vi "Rinocloud_explorer_v0.2.vi"() -> ()   [LabVIEW 2013]
uses:
  Rinocloud_global_variable.vi
panel:
  in  "Extra metadata array":T1(array[cluster])=[{"Attribute"="", "Value"="", "Data type"=enum."<null>"}]
  in  "source ID":string
  in  "destination ID":string
  out "error out":errorcluster
  in  "Active item:":string
  out "RId:":string
  out "OId:":string
  out "FId:":string
  out "DId:":string
  in  "delete":bool
  in  "refresh list":bool
  in  "Tab Control":T2(tab)
  in  "Cluster 2":T3={"Attribute"="Amplitude", "Value"="10", "Data type"=5} {"Data type" items=["Numeric", "String", "1D array of strings", "1D array of doubles", "Data JSON string", "<null>"]}
  in  "Cluster 1":T3={"Attribute"="Amplitude", "Value"="10", "Data type"=5} {"Data type" items=["Numeric", "String", "1D array of strings", "1D array of doubles", "Data JSON string", "<null>"]}
  in  "name":string
  in  "tags":string
  in  "notes":string
  in  "new folder":bool
  in  "upload file":bool
  in  "Name:":string
  in  "Tags:":string
  in  "Notes:":string
  in  "get metadata":bool
  in  "metadata tree":string(tree) caption="Metadata"
  in  "update metadata":bool
  in  "Move":bool
  in  "Destination:":string
  in  "Source:":string
  in  "set source":bool
  in  "set destination":bool
  out "body":string
  out "headers":string
  in  "Active object ID":string
  in  "Active file ID":string
  in  "Active dir ID":string
  in  "Recent ID":string
  in  "menu tree":string(tree) caption="Active path"
  in  "stop":bool
  in  "active child tree":string(tree) caption="File & folder list of the active folder"
  # "Double-click an item to activate"
  # "Custom metadata:"
  # "(tag1,tag2,tag3,...)"
  # "Click the fields to edit"
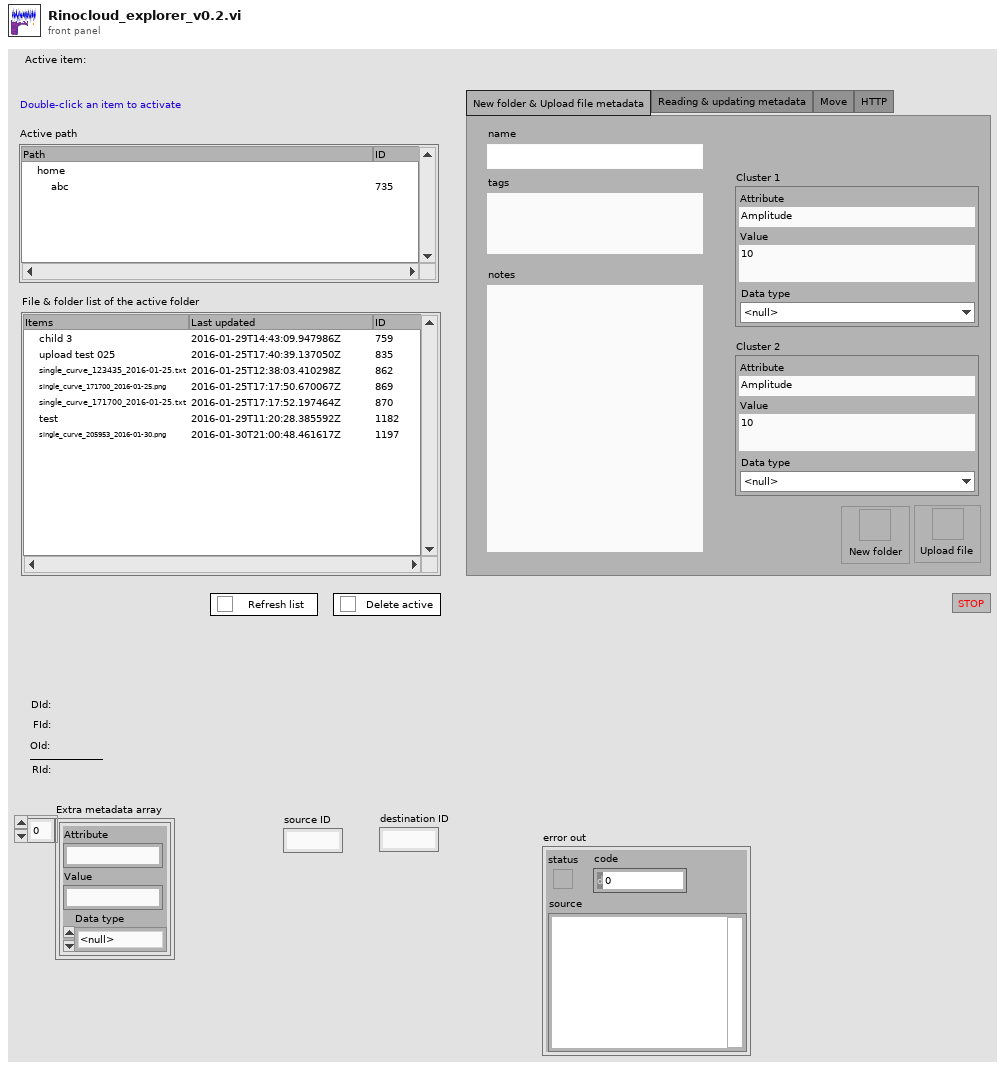
[diagram p1: front panel]
types:
  T1 = cluster{"Attribute":string, "Value":string, "Data type":enum16{"Numeric", "String", "1D array of strings", "1D array of doubles", "Data JSON string", "<null>"}}[]
  T2 = enum32{"New folder & Upload file metadata", "Reading & updating metadata", "Move", "HTTP"}
  T3 = cluster{"Attribute":string, "Value":string, "Data type":u16}
  T4 = cluster{"headers":string, "body":string, "ID":string, "Saved":bool}
  T5 = cluster{"Attribute":string, "Value":string, "Data type":u16}[]
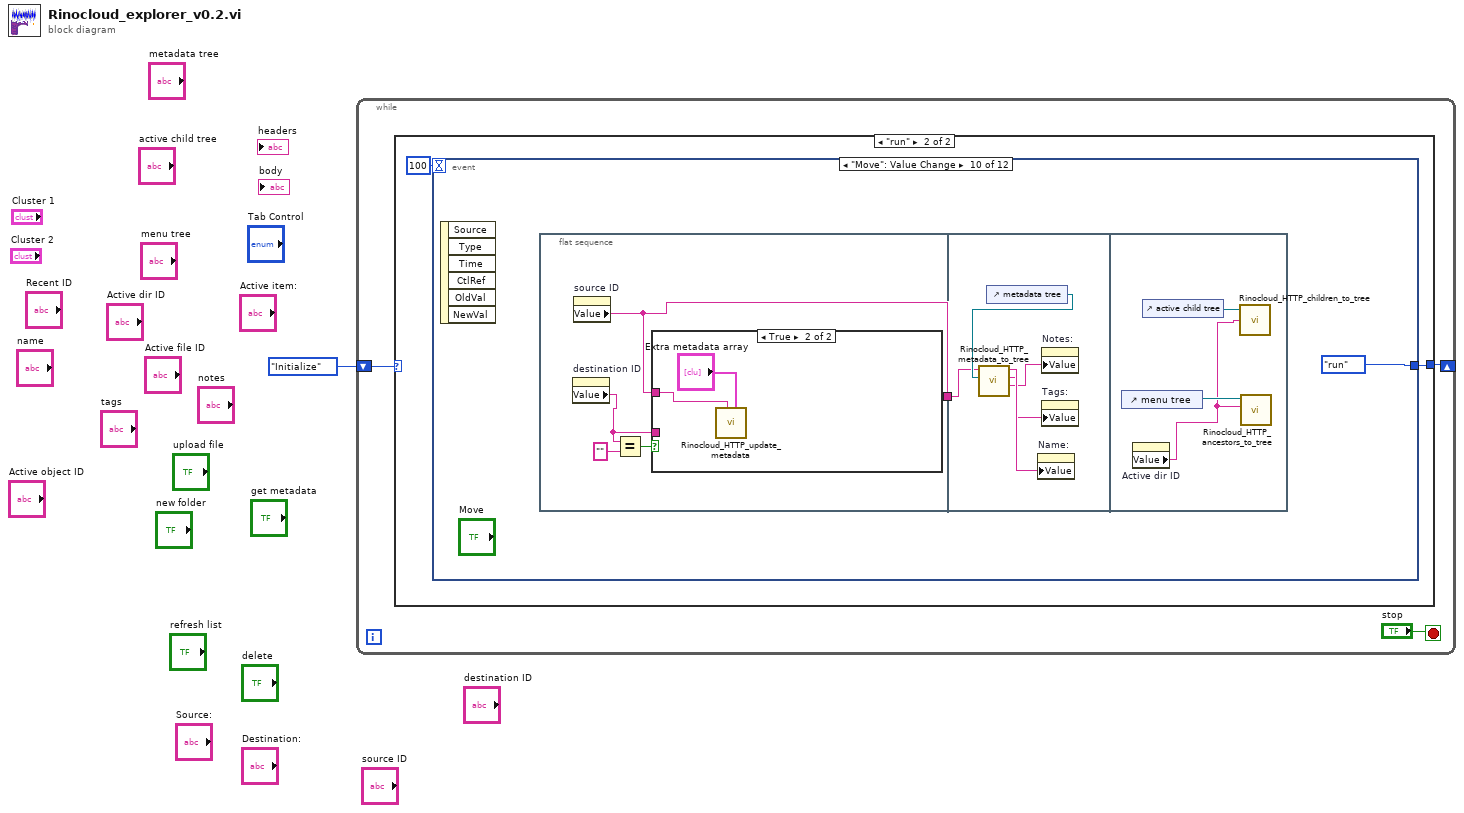
[diagram p0: block diagram]
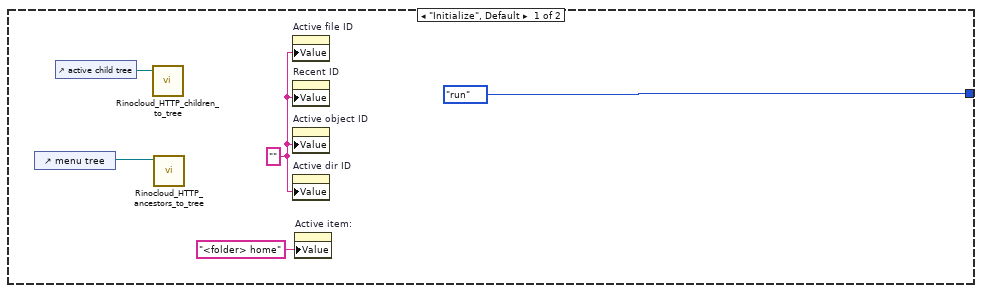
[diagram p2: hidden frame]
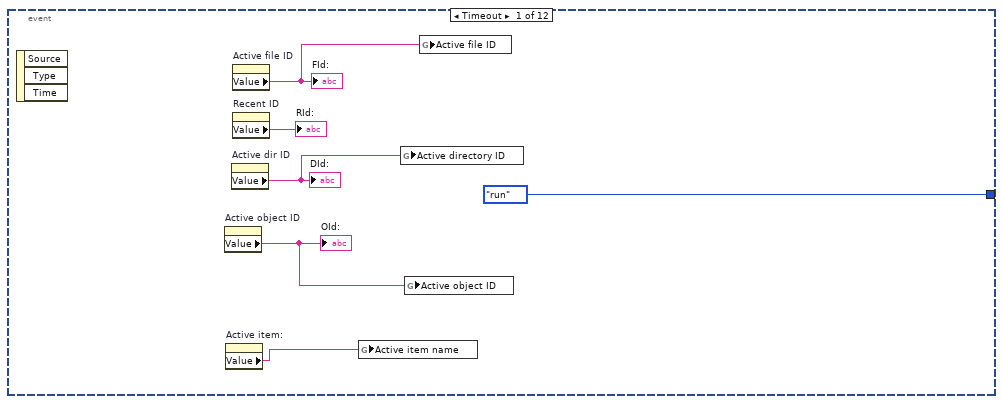
[diagram p3: hidden frame]
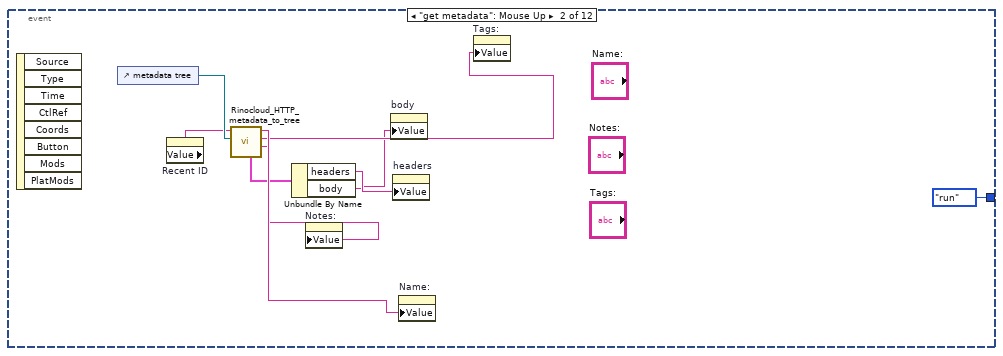
[diagram p4: hidden frame]
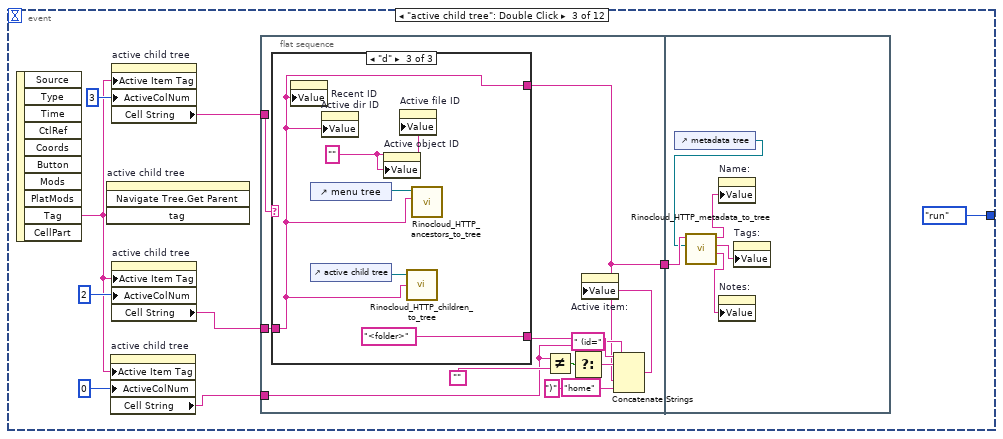
[diagram p5: hidden frame]
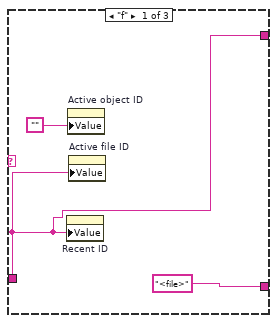
[diagram p6: hidden frame]
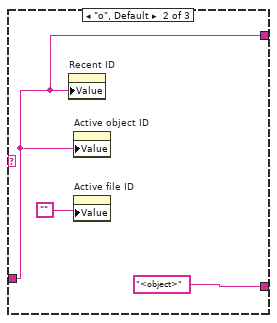
[diagram p7: hidden frame]
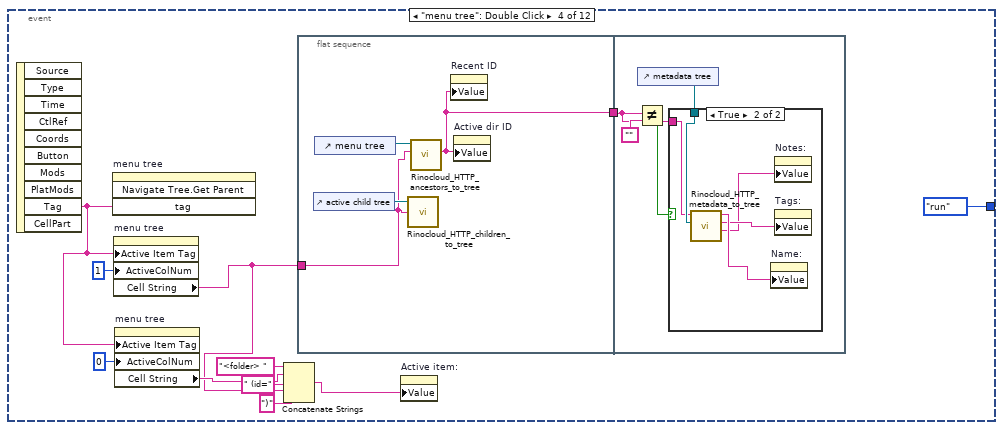
[diagram p8: hidden frame]
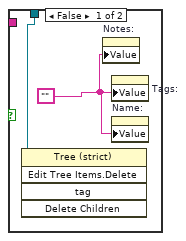
[diagram p9: hidden frame]
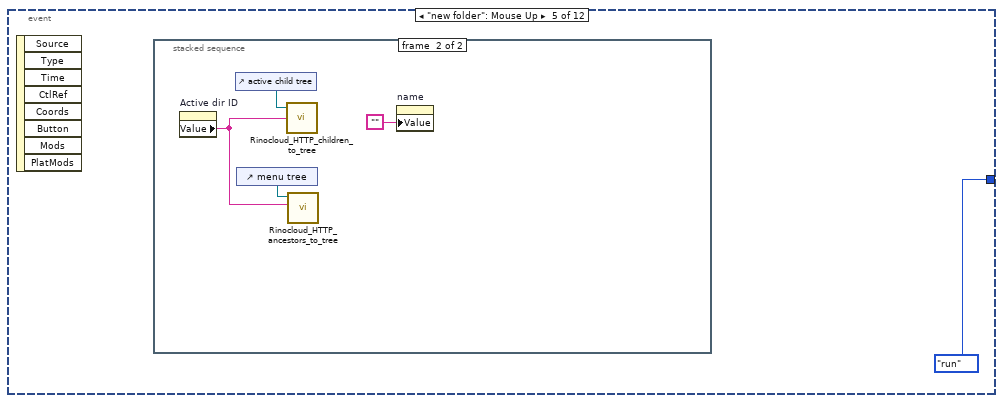
[diagram p10: hidden frame]
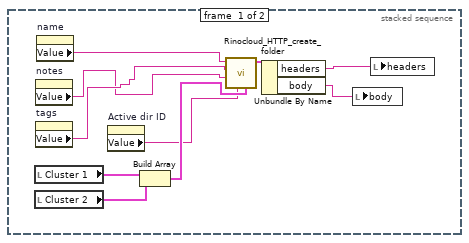
[diagram p11: hidden frame]
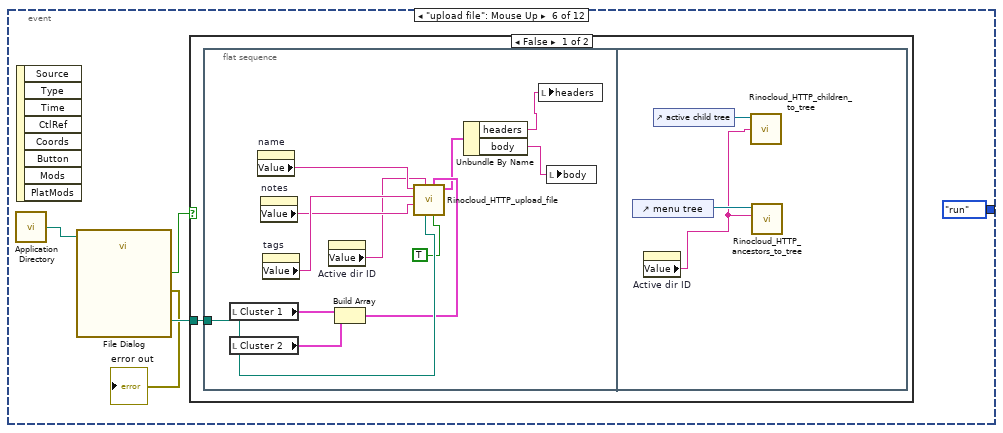
[diagram p12: hidden frame]
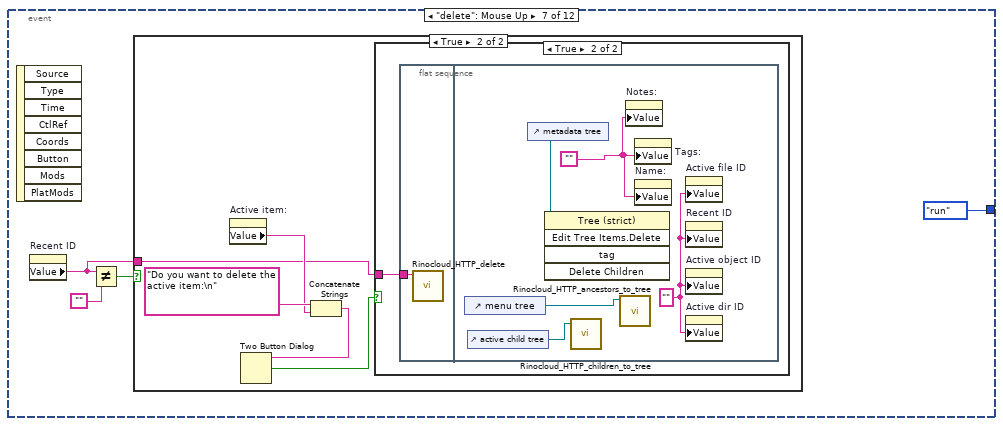
[diagram p14: hidden frame]
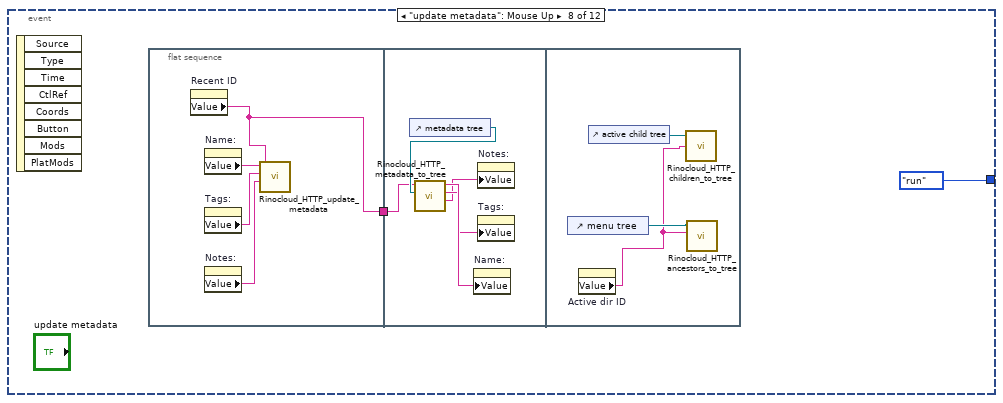
[diagram p17: hidden frame]
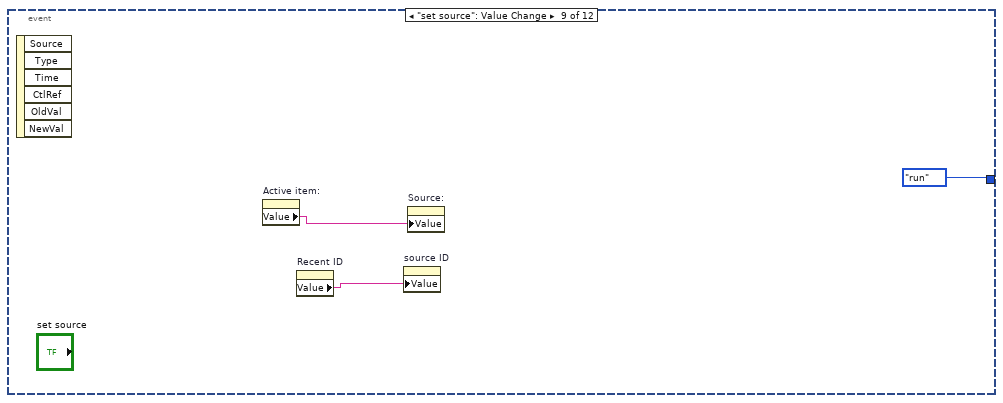
[diagram p18: hidden frame]
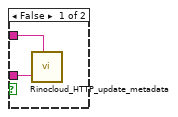
[diagram p19: hidden frame]
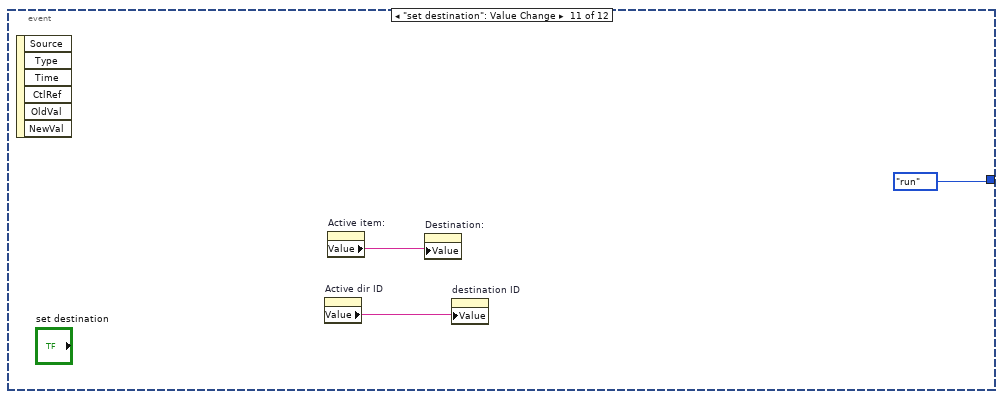
[diagram p20: hidden frame]
diagram:
  n1 = while {
    shift-right: [w3] -> _
    shift-left: enum16{"Initialize"}."Initialize" -> [w4]
    stop <- "stop" stop-if-true
    n2 = case shown="\"run\"" w4 {
      tunnel: [enum16{"Initialize", "run"}."run" w11] -> w3
      frame "Initialize", Default {
        w8 = "" ("Active file ID")
        n3 = control-ref of="menu tree"() -> (w5:refnum<vi>)
        n4 = control-ref of="active child tree"() -> (w6:refnum<vi>)
        n5 = call "Rinocloud_HTTP_children_to_tree.vi"("Tree Ref in"=w6) -> ()  [unwired: 3 in, 2 out]
        n6 = call "Rinocloud_HTTP_ancestors_to_tree.vi"("Tree Ref in"=w5) -> ()  [unwired: 3 in, 4 out]
        n7 = property on="Active file ID" class="Str"("Value"=w8) -> ()  [unwired: 2 in, 2 out]
        n8 = property on="Recent ID" class="Str"("Value"=w8) -> ()  [unwired: 2 in, 2 out]
        n9 = property on="Active object ID" class="Str"("Value"=w8) -> ()  [unwired: 2 in, 2 out]
        n10 = property on="Active dir ID" class="Str"("Value"=w8) -> ()  [unwired: 2 in, 2 out]
        n11 = property on="Active item:" class="Str"("Value"="<folder> home" ("An active item:")) -> ()  [unwired: 2 in, 2 out]
      }
      frame "run" {
        n12 = event shown="[9] \"Move\": Value Change" {
          selector: _ -> [_ _ _ _ _ _ _ _ _ _ _ _]
          dyn-events: _ -> [_ _ _ _ _ _ _ _ _ _ _ _]
          timeout: 100 -> [_ _ _ _ _ _ _ _ _ _ _ _]
          tunnel: [enum16{"Initialize", "run"}."run" enum16{"Initialize", "run"}."run" enum16{"Initialize", "run"}."run" enum16{"Initialize", "run"}."run" enum16{"Initialize", "run"}."run" enum16{"Initialize", "run"}."run" enum16{"Initialize", "run"}."run" enum16{"Initialize", "run"}."run" enum16{"Initialize", "run"}."run" enum16{"Initialize", "run"}."run" enum16{"Initialize", "run"}."run" enum16{"Initialize", "run"}."Initialize"] -> w11
          event Timeout {
            n13 = event-data() -> ()  [unwired: 1 in, 3 out]
            n14 = property on="Active object ID" class="Str"() -> ("Value"=w13:string)  [unwired: 2 in, 2 out]
            "OId:" <- w13
            n15 = property on="Active item:" class="Str"() -> ("Value"=w12:string)  [unwired: 2 in, 2 out]
            n16 = property on="Active dir ID" class="Str"() -> ("Value"=w14:string)  [unwired: 2 in, 2 out]
            "DId:" <- w14
            n17 = property on="Active file ID" class="Str"() -> ("Value"=w15:string)  [unwired: 2 in, 2 out]
            "FId:" <- w15
            n18 = property on="Recent ID" class="Str"() -> ("Value"=→"RId:":string)  [unwired: 2 in, 2 out]
            n19 = global write "Rinocloud_global_variable.vi" "Active item name"(w12) -> ()
            n20 = global write "Rinocloud_global_variable.vi" "Active directory ID"(w14) -> ()
            n21 = global write "Rinocloud_global_variable.vi" "Active object ID"(w13) -> ()
            n22 = global write "Rinocloud_global_variable.vi" "Active file ID"(w15) -> ()
          }
          event "get metadata": Mouse Up {
            n23 = event-data() -> ()  [unwired: 1 in, 8 out]
            n24 = control-ref of="metadata tree"() -> (w25:refnum<vi>)
            n25 = property on="Recent ID" class="Str"() -> ("Value"=w24:string)  [unwired: 2 in, 2 out]
            n26 = call "Rinocloud_HTTP_metadata_to_tree.vi"("JSON Tree Expanded Reference"=w25, "id"=w24) -> ("Notes"=w21:string, "Tags"=w22:string, "Name"=w23:string, "Status"=w20:T4)  [unwired: 4 in, 2 out]
            n27 = Unbundle By Name(w20) -> ("headers"=w19:string, "body"=w18:string)
            n28 = property on="Notes:" class="Str"("Value"=w21) -> ()  [unwired: 2 in, 2 out]
            n29 = property on="body" class="Str"("Value"=w18) -> ()  [unwired: 2 in, 2 out]
            n30 = property on="headers" class="Str"("Value"=w19) -> ()  [unwired: 2 in, 2 out]
            n31 = property on="Name:" class="Str"("Value"=w23) -> ()  [unwired: 2 in, 2 out]
            n32 = property on="Tags:" class="Str"("Value"=w22) -> ()  [unwired: 2 in, 2 out]
          }
          event "active child tree": Double Click {
            n33 = event-data() -> ("Tag"=w30:string)  [unwired: 1 in, 9 out]
            n34 = invoke on="active child tree" class="Tree (strict)" method="Navigate Tree.Get Parent"("tag"=w30) -> ()  [unwired: 3 in, 4 out]
            n35 = property on="active child tree" class="Tree (strict)"("Active Item Tag"=w30, "ActiveColNum"=0 ("Active Cell:Active Column Number")) -> ("Cell String"=w28:string)  [unwired: 2 in, 2 out]
            n36 = property on="active child tree" class="Tree (strict)"("Active Item Tag"=w30, "ActiveColNum"=3 ("Active Cell:Active Column Number")) -> ("Cell String"=w31:string)  [unwired: 2 in, 2 out]
            n37 = property on="active child tree" class="Tree (strict)"("Active Item Tag"=w30, "ActiveColNum"=2 ("Active Cell:Active Column Number")) -> ("Cell String"=w33:string)  [unwired: 2 in, 2 out]
            n38 = flat-sequence {
              tunnel: w33 -> [w47]
              tunnel: w31 -> [w46]
              tunnel: w28 -> [w42]
              tunnel: [w36] -> w27
              tunnel: w27 -> [w63]
              frame #0 {
                n39 = case shown="\"d\"" w46 {
                  tunnel: w47 -> [w48 w51 w54]
                  tunnel: ["<file>" ("f") "<object>" ("f") "<folder>" ("f")] -> w41
                  tunnel: [w48 w51 w54] -> w36
                  frame "f" {
                    n40 = property on="Recent ID" class="Str"("Value"=w48) -> ()  [unwired: 2 in, 2 out]
                    n41 = property on="Active object ID" class="Str"("Value"="") -> ()  [unwired: 2 in, 2 out]
                    n42 = property on="Active file ID" class="Str"("Value"=w48) -> ()  [unwired: 2 in, 2 out]
                  }
                  frame "o", Default {
                    n43 = property on="Recent ID" class="Str"("Value"=w51) -> ()  [unwired: 2 in, 2 out]
                    n44 = property on="Active object ID" class="Str"("Value"=w51) -> ()  [unwired: 2 in, 2 out]
                    n45 = property on="Active file ID" class="Str"("Value"="") -> ()  [unwired: 2 in, 2 out]
                  }
                  frame "d" {
                    w58 = "" ("Active file ID")
                    n46 = property on="Recent ID" class="Str"("Value"=w54) -> ()  [unwired: 2 in, 2 out]
                    n47 = control-ref of="menu tree"() -> (w55:refnum<vi>)
                    n48 = control-ref of="active child tree"() -> (w56:refnum<vi>)
                    n49 = property on="Active dir ID" class="Str"("Value"=w54) -> ()  [unwired: 2 in, 2 out]
                    n50 = property on="Active object ID" class="Str"("Value"=w58) -> ()  [unwired: 2 in, 2 out]
                    n51 = property on="Active file ID" class="Str"("Value"=w58) -> ()  [unwired: 2 in, 2 out]
                    n52 = call "Rinocloud_HTTP_children_to_tree.vi"("id"=w54, "Tree Ref in"=w56) -> ()  [unwired: 2 in, 2 out]
                    n53 = call "Rinocloud_HTTP_ancestors_to_tree.vi"("id"=w54, "Tree Ref in"=w55) -> ()  [unwired: 2 in, 4 out]
                  }
                }
                n54 = Not Equal?(x=w42, y="") -> (x != y?=w44:bool)
                n55 = Select(t=w42, s=w44, f="home") -> (s? t:f=w40:string)
                n56 = Concatenate Strings(w41, w40, " (id=" ("string"), w36, ")" ("string")) -> (w39:string)
                n57 = property on="Active item:" class="Str"("Value"=w39) -> ()  [unwired: 2 in, 2 out]
              }
              frame #1 {
                n58 = control-ref of="metadata tree"() -> (w62:refnum<vi>)
                n59 = call "Rinocloud_HTTP_metadata_to_tree.vi"("JSON Tree Expanded Reference"=w62, "id"=w63) -> ("Notes"=w61:string, "Tags"=w60:string, "Name"=w59:string)  [unwired: 4 in, 3 out]
                n60 = property on="Name:" class="Str"("Value"=w59) -> ()  [unwired: 2 in, 2 out]
                n61 = property on="Notes:" class="Str"("Value"=w61) -> ()  [unwired: 2 in, 2 out]
                n62 = property on="Tags:" class="Str"("Value"=w60) -> ()  [unwired: 2 in, 2 out]
              }
            }
          }
          event "menu tree": Double Click {
            n63 = event-data() -> ("Tag"=w72:string)  [unwired: 1 in, 9 out]
            n64 = invoke on="menu tree" class="Tree (strict)" method="Navigate Tree.Get Parent"("tag"=w72) -> ()  [unwired: 3 in, 4 out]
            n65 = property on="menu tree" class="Tree (strict)"("Active Item Tag"=w72, "ActiveColNum"=1 ("Active Cell:Active Column Number")) -> ("Cell String"=w67:string)  [unwired: 2 in, 2 out]
            n66 = property on="menu tree" class="Tree (strict)"("Active Item Tag"=w72, "ActiveColNum"=0 ("Active Cell:Active Column Number")) -> ("Cell String"=w68:string)  [unwired: 2 in, 2 out]
            n67 = Concatenate Strings("<folder> " ("string"), w68, " (id=" ("string"), w67, ")" ("string")) -> (w64:string)
            n68 = flat-sequence {
              tunnel: w67 -> [w75]
              tunnel: [w78] -> w70
              tunnel: w70 -> [w80]
              frame #0 {
                n69 = control-ref of="active child tree"() -> (w77:refnum<vi>)
                n70 = control-ref of="menu tree"() -> (w76:refnum<vi>)
                n71 = call "Rinocloud_HTTP_children_to_tree.vi"("id"=w75, "Tree Ref in"=w77) -> ()  [unwired: 2 in, 2 out]
                n72 = call "Rinocloud_HTTP_ancestors_to_tree.vi"("id"=w75, "Tree Ref in"=w76) -> ("last ID"=w78:string)  [unwired: 2 in, 3 out]
                n73 = property on="Recent ID" class="Str"("Value"=w78) -> ()  [unwired: 2 in, 2 out]
                n74 = property on="Active dir ID" class="Str"("Value"=w78) -> ()  [unwired: 2 in, 2 out]
              }
              frame #1 {
                n75 = Not Equal?(x=w80, y="") -> (x != y?=w81:bool)
                n76 = control-ref of="metadata tree"() -> (w79:refnum<vi>)
                n77 = case shown="True" w81 {
                  tunnel: w80 -> [_ w88]
                  tunnel: w79 -> [w83 w89]
                  frame False {
                    w84 = ""
                    n78 = invoke class="Tree (strict)" method="Edit Tree Items.Delete"(reference=w83) -> ()  [unwired: 4 in, 5 out]
                    n79 = property on="Notes:" class="Str"("Value"=w84) -> ()  [unwired: 2 in, 2 out]
                    n80 = property on="Tags:" class="Str"("Value"=w84) -> ()  [unwired: 2 in, 2 out]
                    n81 = property on="Name:" class="Str"("Value"=w84) -> ()  [unwired: 2 in, 2 out]
                  }
                  frame True {
                    n82 = call "Rinocloud_HTTP_metadata_to_tree.vi"("JSON Tree Expanded Reference"=w89, "id"=w88) -> ("Notes"=w85:string, "Tags"=w86:string, "Name"=w87:string)  [unwired: 4 in, 3 out]
                    n83 = property on="Name:" class="Str"("Value"=w87) -> ()  [unwired: 2 in, 2 out]
                    n84 = property on="Notes:" class="Str"("Value"=w85) -> ()  [unwired: 2 in, 2 out]
                    n85 = property on="Tags:" class="Str"("Value"=w86) -> ()  [unwired: 2 in, 2 out]
                  }
                }
              }
            }
            n86 = property on="Active item:" class="Str"("Value"=w64) -> ()  [unwired: 2 in, 2 out]
          }
          event "new folder": Mouse Up {
            n87 = event-data() -> ()  [unwired: 1 in, 8 out]
            n88 = stacked-sequence {
              frame #0 {
                n89 = local read "Cluster 1"() -> (w100:T3)
                n90 = local read "Cluster 2"() -> (w99:T3)
                n91 = property on="notes" class="Str"() -> ("Value"=w96:string)  [unwired: 2 in, 2 out]
                n92 = property on="tags" class="Str"() -> ("Value"=w97:string)  [unwired: 2 in, 2 out]
                n93 = property on="name" class="Str"() -> ("Value"=w98:string)  [unwired: 2 in, 2 out]
                n94 = property on="Active dir ID" class="Str"() -> ("Value"=w94:string)  [unwired: 2 in, 2 out]
                n95 = Build Array(w100, w99) -> (w95:T5)
                n96 = call "Rinocloud_HTTP_create_folder.vi"("Extra metadata array"=w95, "Parent ID"=w94, "Notes"=w96, "Tags"=w97, "Name"=w98) -> ("Status"=w93:T4)  [unwired: 3 in, 1 out]
                n97 = Unbundle By Name(w93) -> ("headers"=w92:string, "body"=w91:string)
                n98 = local write "body"(w91) -> ()
                n99 = local write "headers"(w92) -> ()
              }
              frame #1 {
                n100 = property on="Active dir ID" class="Str"() -> ("Value"=w101:string)  [unwired: 2 in, 2 out]
                n101 = control-ref of="active child tree"() -> (w103:refnum<vi>)
                n102 = control-ref of="menu tree"() -> (w102:refnum<vi>)
                n103 = call "Rinocloud_HTTP_children_to_tree.vi"("id"=w101, "Tree Ref in"=w103) -> ()  [unwired: 2 in, 2 out]
                n104 = call "Rinocloud_HTTP_ancestors_to_tree.vi"("id"=w101, "Tree Ref in"=w102) -> ()  [unwired: 2 in, 4 out]
                n105 = property on="name" class="Str"("Value"="") -> ()  [unwired: 2 in, 2 out]
              }
            }
          }
          event "upload file": Mouse Up {
            n106 = call <vilib>:"Application Directory.vi"() -> ("Application Directory"=w108:path)
            n107 = event-data() -> ()  [unwired: 1 in, 8 out]
            n108 = call "File Dialog"("start path"=w108) -> ("selected path"=w106:path, "cancelled"=w107:bool, "error out"=→"error out":errorcluster)  [unwired: 11 in, 1 out]
            n109 = case shown="False" w107 {
              tunnel: w106 -> [w110 _]
              frame False {
                n110 = flat-sequence {
                  tunnel: w110 -> [w120]
                  frame #0 {
                    n111 = local read "Cluster 1"() -> (w122:T3)
                    n112 = local read "Cluster 2"() -> (w121:T3)
                    n113 = property on="name" class="Str"() -> ("Value"=w118:string)  [unwired: 2 in, 2 out]
                    n114 = property on="notes" class="Str"() -> ("Value"=w116:string)  [unwired: 2 in, 2 out]
                    n115 = property on="tags" class="Str"() -> ("Value"=w117:string)  [unwired: 2 in, 2 out]
                    n116 = property on="Active dir ID" class="Str"() -> ("Value"=w115:string)  [unwired: 2 in, 2 out]
                    n117 = Build Array(w122, w121) -> (w114:T5)
                    n118 = call "Rinocloud_HTTP_upload_file.vi"("Store locally"=TRUE, "Extra metadata array"=w114, "Path in"=w120, "Parent ID"=w115, "Notes"=w116, "Tags"=w117, "Name"=w118) -> ("Status"=w113:T4)  [unwired: 2 in, 2 out]
                    n119 = Unbundle By Name(w113) -> ("headers"=w112:string, "body"=w111:string)
                    n120 = local write "headers"(w112) -> ()
                    n121 = local write "body"(w111) -> ()
                  }
                  frame #1 {
                    n122 = control-ref of="menu tree"() -> (w124:refnum<vi>)
                    n123 = property on="Active dir ID" class="Str"() -> ("Value"=w123:string)  [unwired: 2 in, 2 out]
                    n124 = control-ref of="active child tree"() -> (w125:refnum<vi>)
                    n125 = call "Rinocloud_HTTP_children_to_tree.vi"("id"=w123, "Tree Ref in"=w125) -> ()  [unwired: 2 in, 2 out]
                    n126 = call "Rinocloud_HTTP_ancestors_to_tree.vi"("id"=w123, "Tree Ref in"=w124) -> ()  [unwired: 2 in, 4 out]
                  }
                }
              }
              frame True {
              }
            }
          }
          event "delete": Mouse Up {
            n127 = event-data() -> ()  [unwired: 1 in, 8 out]
            n128 = property on="Recent ID" class="Str"() -> ("Value"=w126:string)  [unwired: 2 in, 2 out]
            n129 = Not Equal?(x=w126, y="") -> (x != y?=w128:bool)
            n130 = case shown="True" w128 {
              tunnel: w126 -> [_ w130]
              frame False {
              }
              frame True {
                n131 = property on="Active item:" class="Str"() -> ("Value"=w131:string)  [unwired: 2 in, 2 out]
                n132 = Concatenate Strings("Do you want to delete the active item:\n" ("message"), w131) -> (w133:string)
                n133 = Two Button Dialog(message=w133) -> (T button?=w132:bool)  [unwired: 2 in]
                n134 = case shown="True" w132 {
                  tunnel: w130 -> [_ w135]
                  frame False {
                  }
                  frame True {
                    n135 = flat-sequence {
                      tunnel: w135 -> [w136]
                      frame #0 {
                        n136 = call "Rinocloud_HTTP_delete.vi"("ID"=w136) -> ()  [unwired: 6 in, 2 out]
                      }
                      frame #1 {
                        w139 = ""
                        w141 = "" ("Active file ID")
                        n137 = control-ref of="menu tree"() -> (w137:refnum<vi>)
                        n138 = control-ref of="active child tree"() -> (w138:refnum<vi>)
                        n139 = control-ref of="metadata tree"() -> (w140:refnum<vi>)
                        n140 = invoke class="Tree (strict)" method="Edit Tree Items.Delete"(reference=w140) -> ()  [unwired: 4 in, 5 out]
                        n141 = call "Rinocloud_HTTP_children_to_tree.vi"("Tree Ref in"=w138) -> ()  [unwired: 3 in, 2 out]
                        n142 = call "Rinocloud_HTTP_ancestors_to_tree.vi"("Tree Ref in"=w137) -> ()  [unwired: 3 in, 4 out]
                        n143 = property on="Notes:" class="Str"("Value"=w139) -> ()  [unwired: 2 in, 2 out]
                        n144 = property on="Tags:" class="Str"("Value"=w139) -> ()  [unwired: 2 in, 2 out]
                        n145 = property on="Name:" class="Str"("Value"=w139) -> ()  [unwired: 2 in, 2 out]
                        n146 = property on="Active file ID" class="Str"("Value"=w141) -> ()  [unwired: 2 in, 2 out]
                        n147 = property on="Recent ID" class="Str"("Value"=w141) -> ()  [unwired: 2 in, 2 out]
                        n148 = property on="Active object ID" class="Str"("Value"=w141) -> ()  [unwired: 2 in, 2 out]
                        n149 = property on="Active dir ID" class="Str"("Value"=w141) -> ()  [unwired: 2 in, 2 out]
                      }
                    }
                  }
                }
              }
            }
          }
          event "update metadata": Mouse Up {
            n150 = event-data() -> ()  [unwired: 1 in, 8 out]
            n151 = flat-sequence {
              tunnel: [w144] -> w142
              tunnel: w142 -> [w151]
              frame #0 {
                n152 = property on="Recent ID" class="Str"() -> ("Value"=w144:string)  [unwired: 2 in, 2 out]
                n153 = property on="Name:" class="Str"() -> ("Value"=w145:string)  [unwired: 2 in, 2 out]
                n154 = property on="Tags:" class="Str"() -> ("Value"=w147:string)  [unwired: 2 in, 2 out]
                n155 = property on="Notes:" class="Str"() -> ("Value"=w146:string)  [unwired: 2 in, 2 out]
                n156 = call "Rinocloud_HTTP_update_metadata.vi"("self ID"=w144, "Notes"=w146, "Tags"=w147, "Name"=w145) -> ()  [unwired: 6 in, 2 out]
              }
              frame #1 {
                n157 = control-ref of="metadata tree"() -> (w152:refnum<vi>)
                n158 = call "Rinocloud_HTTP_metadata_to_tree.vi"("JSON Tree Expanded Reference"=w152, "id"=w151) -> ("Notes"=w148:string, "Tags"=w149:string, "Name"=w150:string)  [unwired: 4 in, 3 out]
                n159 = property on="Name:" class="Str"("Value"=w150) -> ()  [unwired: 2 in, 2 out]
                n160 = property on="Notes:" class="Str"("Value"=w148) -> ()  [unwired: 2 in, 2 out]
                n161 = property on="Tags:" class="Str"("Value"=w149) -> ()  [unwired: 2 in, 2 out]
              }
              frame #2 {
                n162 = control-ref of="menu tree"() -> (w154:refnum<vi>)
                n163 = property on="Active dir ID" class="Str"() -> ("Value"=w153:string)  [unwired: 2 in, 2 out]
                n164 = control-ref of="active child tree"() -> (w155:refnum<vi>)
                n165 = call "Rinocloud_HTTP_children_to_tree.vi"("id"=w153, "Tree Ref in"=w155) -> ()  [unwired: 2 in, 2 out]
                n166 = call "Rinocloud_HTTP_ancestors_to_tree.vi"("id"=w153, "Tree Ref in"=w154) -> ()  [unwired: 2 in, 4 out]
              }
            }
          }
          event "set source": Value Change {
            n167 = event-data() -> ()  [unwired: 1 in, 6 out]
            n168 = property on="Active item:" class="Str"() -> ("Value"=w157:string)  [unwired: 2 in, 2 out]
            n169 = property on="Recent ID" class="Str"() -> ("Value"=w158:string)  [unwired: 2 in, 2 out]
            n170 = property on="source ID" class="Str"("Value"=w158) -> ()  [unwired: 2 in, 2 out]
            n171 = property on="Source:" class="Str"("Value"=w157) -> ()  [unwired: 2 in, 2 out]
          }
          event "Move": Value Change {
            n172 = event-data() -> ()  [unwired: 1 in, 6 out]
            n173 = flat-sequence {
              tunnel: [w162] -> w160
              tunnel: w160 -> [w172]
              frame #0 {
                n174 = property on="destination ID" class="Str"() -> ("Value"=w161:string)  [unwired: 2 in, 2 out]
                n175 = property on="source ID" class="Str"() -> ("Value"=w162:string)  [unwired: 2 in, 2 out]
                n176 = Equal?(x=w161, y="") -> (x = y?=w163:bool)
                n177 = case shown="True" w163 {
                  tunnel: w162 -> [w166 w167]
                  tunnel: w161 -> [w165 _]
                  frame False {
                    n178 = call "Rinocloud_HTTP_update_metadata.vi"("parent ID"=w165, "self ID"=w166) -> ()  [unwired: 8 in, 2 out]
                  }
                  frame True {
                    n179 = call "Rinocloud_HTTP_update_metadata.vi"("Extra metadata array"="Extra metadata array", "self ID"=w167) -> ()  [unwired: 8 in, 2 out]
                  }
                }
              }
              frame #1 {
                n180 = control-ref of="metadata tree"() -> (w173:refnum<vi>)
                n181 = call "Rinocloud_HTTP_metadata_to_tree.vi"("JSON Tree Expanded Reference"=w173, "id"=w172) -> ("Notes"=w169:string, "Tags"=w170:string, "Name"=w171:string)  [unwired: 4 in, 3 out]
                n182 = property on="Name:" class="Str"("Value"=w171) -> ()  [unwired: 2 in, 2 out]
                n183 = property on="Notes:" class="Str"("Value"=w169) -> ()  [unwired: 2 in, 2 out]
                n184 = property on="Tags:" class="Str"("Value"=w170) -> ()  [unwired: 2 in, 2 out]
              }
              frame #2 {
                n185 = control-ref of="menu tree"() -> (w175:refnum<vi>)
                n186 = property on="Active dir ID" class="Str"() -> ("Value"=w174:string)  [unwired: 2 in, 2 out]
                n187 = control-ref of="active child tree"() -> (w176:refnum<vi>)
                n188 = call "Rinocloud_HTTP_children_to_tree.vi"("id"=w174, "Tree Ref in"=w176) -> ()  [unwired: 2 in, 2 out]
                n189 = call "Rinocloud_HTTP_ancestors_to_tree.vi"("id"=w174, "Tree Ref in"=w175) -> ()  [unwired: 2 in, 4 out]
              }
            }
          }
          event "set destination": Value Change {
            n190 = event-data() -> ()  [unwired: 1 in, 6 out]
            n191 = property on="Active dir ID" class="Str"() -> ("Value"=w178:string)  [unwired: 2 in, 2 out]
            n192 = property on="Active item:" class="Str"() -> ("Value"=w179:string)  [unwired: 2 in, 2 out]
            n193 = property on="Destination:" class="Str"("Value"=w179) -> ()  [unwired: 2 in, 2 out]
            n194 = property on="destination ID" class="Str"("Value"=w178) -> ()  [unwired: 2 in, 2 out]
          }
          event "refresh list": Mouse Up {
            n195 = event-data() -> ()  [unwired: 1 in, 8 out]
          }
        }
      }
    }
  }
